vi "Show ALL Front Panel Objects.vi"(2 "error in (no error)":errorcluster, 3 "Stop Calling VI? (T)":bool=TRUE) -> (0 "error out":errorcluster, 1 "VI has Tab Control(s)?":bool)   [LabVIEW 2014]
doc: "Place this subVI in the block diagram of a VI whose front panel objects you wish to make visible. This will even make Tab Controls and the objects they contain unhidden. \n\nIf the Stop Callin VI? Control is true, it will abort the VIs and stop LabVIEW after this VI has finished executing. Set this to false if you plan on using it as an initialization step every time you run the calling VI."
panel:
  # "Place this subVI in the block diagram of a VI whose front panel objects you wish to make visible.  This will even make Tab Controls and the objects they contain unhidden.\n\nIf the Stop Calling VI? Control is true, it will abort the calling VI after the controls have been made visiable"
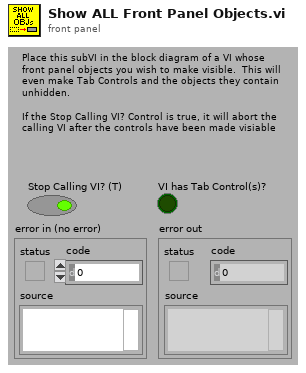
[diagram p1: front panel]
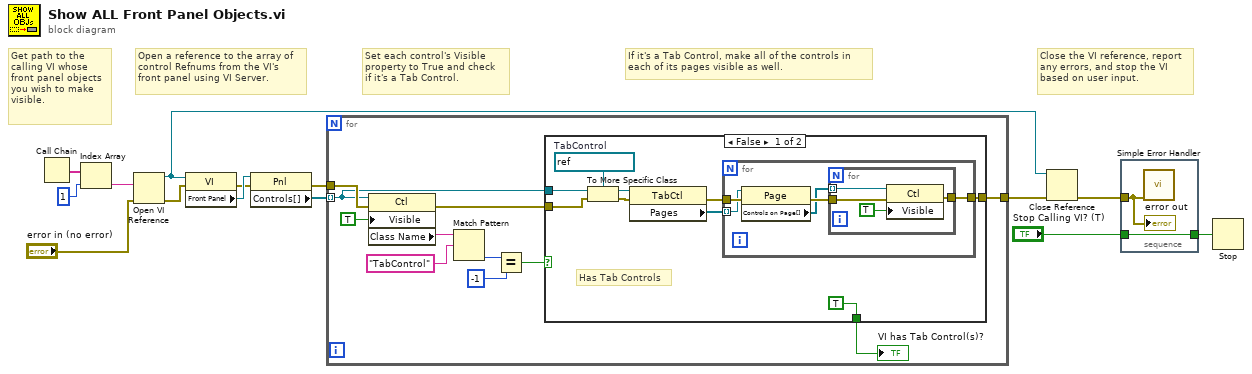
[diagram p0: block diagram]
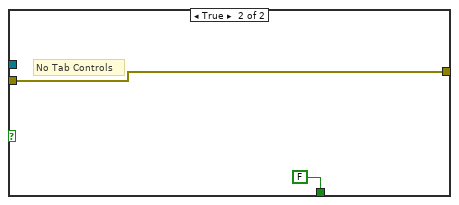
[diagram p2: hidden frame]
diagram:
  # "Close the VI reference, report\nany errors, and stop the VI \nbased on user input."
  # "If it's a Tab Control, make all of the controls in\neach of its pages visible as well."
  # "Set each control's Visible \nproperty to True and check\nif it's a Tab Control."
  # "Open a reference to the array of\ncontrol Refnums from the VI's\nfront panel using VI Server."
  # "Get path to the \ncalling VI whose \nfront panel objects\nyou wish to make \nvisible."
  n1 = Call Chain() -> (call chain=w11:string[])
  n2 = Index Array(array=w11, index=1) -> (element=w1:string)
  n3 = Open VI Reference(vi path=w1, error in (no error)="error in (no error)") -> (vi reference=w2:refnum<vi>, error out=w13:errorcluster)  [unwired: 4 in]
  n4 = property class="VI"(reference=w2, error in=w13) -> (error out=w12:errorcluster, "Front Panel"=w14:refnum<vi>)  [unwired: 1 out]
  n5 = property class="Pnl"(reference=w14, error in=w12) -> (error out=w9:errorcluster, "Controls[]"=w8:refnum<vi>[])  [unwired: 1 out]
  n6 = for {
    tunnel: w8 -> [w18] mode=indexing
    tunnel: w9 -> [w24]
    tunnel: [w16] -> w4
    n7 = property class="Ctl"(reference=w18, error in=w24, "Visible"=TRUE) -> (error out=w17:errorcluster, "Class Name"=w23:string)  [unwired: 1 out]
    n8 = Match Pattern(string=w23, regular expression="TabControl") -> (offset past match=w21:i32)  [unwired: 1 in, 3 out]
    n9 = Equal?(x=w21, y=-1) -> (x = y?=w19:bool)
    n10 = case shown="False" w19 {
      tunnel: w18 -> [w34 _]
      tunnel: w17 -> [w32 w44]
      tunnel: [TRUE ("Visible") FALSE ("Visible")] -> w15
      tunnel: [w26 w44] -> w16
      frame False {
        w33 = refnum<vi> refnum  # TabControl
        # "Has Tab Controls"
        n11 = To More Specific Class(target class=w33, reference=w34, error in=w32) -> (specific class reference=w31:refnum<vi>, error out=w30:errorcluster)
        n12 = property class="TabCtl"(reference=w31, error in=w30) -> (error out=w29:errorcluster, "Pages"=w28:refnum<vi>[])  [unwired: 1 out]
        n13 = for {
          tunnel: w29 -> [w39]
          tunnel: w28 -> [w38] mode=indexing
          tunnel: [w35] -> w26
          n14 = property class="Page"(reference=w38, error in=w39) -> (error out=w37:errorcluster, "Controls on Page[]"=w36:refnum<vi>[])  [unwired: 1 out]
          n15 = for {
            tunnel: w37 -> [w43]
            tunnel: w36 -> [w42] mode=indexing
            tunnel: [w40] -> w35
            n16 = property class="Ctl"(reference=w42, error in=w43, "Visible"=TRUE) -> (error out=w40:errorcluster)  [unwired: 1 out]
          }
        }
      }
      frame True {
        # "No Tab Controls"
      }
    }
    "VI has Tab Control(s)?" <- w15
  }
  n17 = Close Reference(reference=w2, error in (no error)=w4) -> (error out=w7:errorcluster)
  n18 = stacked-sequence {
    tunnel: "Stop Calling VI? (T)" -> [w47]
    tunnel: w7 -> [w46]
    tunnel: [w47] -> w5
    frame #0 {
      n19 = call <vilib>:"Simple Error Handler.vi"("error in (no error)"=w46) -> ()  [unwired: 4 in, 5 out]
      "error out" <- w46
    }
  }
  n20 = Stop(stop? (T)=w5) -> ()
